vi "UE9 eDAC Example.vi"() -> (0 "error out":errorcluster)   [LabVIEW 2021]
panel:
  in  "Address":string="192.168.1.209"
  in  "ConnectionType":u16(ring) items=["LJ_ctUSB", "LJ_ctETHERNET"]
  in  "FirstFound":bool=TRUE
  in  "Channel":i32
  out "Error Message":string
  in  "Voltage":dbl format="%.3f"
  # "Sets 1 analog output using the UD easy function eDAC."
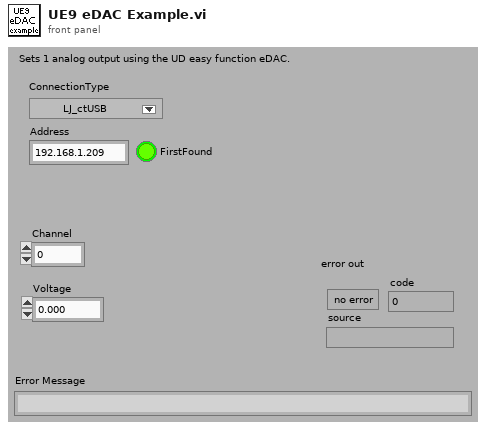
[diagram p1: front panel]
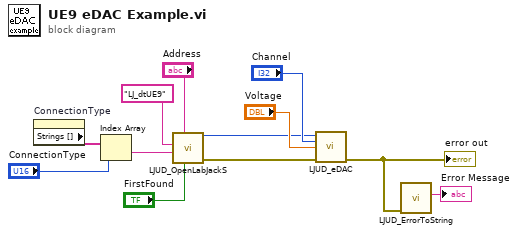
[diagram p0: block diagram]
diagram:
  n1 = property on="ConnectionType" class="Ring (strict)"() -> ("Strings []"=w8:string[])  [unwired: 2 in, 2 out]
  n2 = Index Array(array=w8, index="ConnectionType") -> (element=w4:string)
  n3 = call "LJUD_OpenLabJackS.vi"("FirstFound"="FirstFound", "Address"="Address", "ConnectionType"=w4, "DeviceType"="LJ_dtUE9") -> ("error out"=w1:errorcluster, "Handle"=w2:i32)  [unwired: 5 in, 1 out]
  n4 = call "LJUD_eDAC.vi"("Handle In"=w2, "Channel"="Channel", "Voltage"="Voltage", "error in"=w1) -> ("error out"=w11:errorcluster)  [unwired: 10 in, 1 out]
  "error out" <- w11
  n5 = call "LJUD_ErrorToString.vi"("error in"=w11) -> ("String"=→"Error Message":string)  [unwired: 10 in]
